vi "append at intervals.vi"(6 "Log Period [s]":dbl=10.0, 8 "error in (no error)":errorcluster, 9 "Array":dbl[](array[numeric]), 10 "Previous Time":timestamp, 11 "Data Log":refnum<class "data log.lvclass">) -> (0 "error constant":errorcluster, 2 "New Previous Time":timestamp, 3 "data log out":refnum<class "data log.lvclass">)   [LabVIEW 2025, in "data log.lvclass"]
uses:
  data log.lvclass
  data log.lvclass/data log.ctl
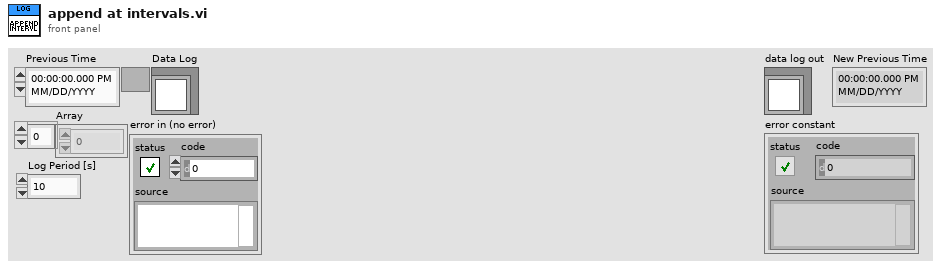
[diagram p1: front panel]
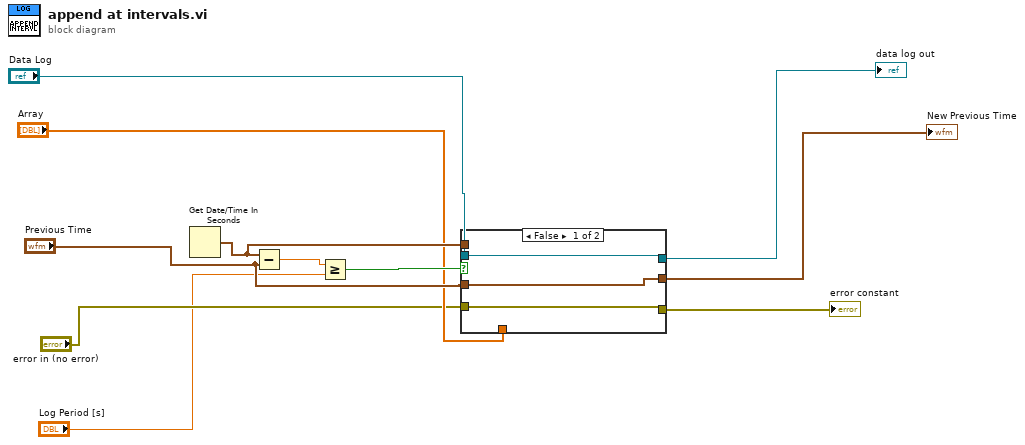
[diagram p0: block diagram]
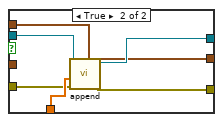
[diagram p2: hidden frame]
diagram:
  n1 = Get Date/Time In Seconds() -> (seconds since 1Jan1904=w9:timestamp)
  n2 = Subtract(x=w9, y="Previous Time") -> (x-y=w11:dbl)
  n3 = Greater Or Equal?(x=w11, y="Log Period [s]") -> (x >= y?=w10:bool)
  n4 = case shown="False" w10 {
    tunnel: [w14 w20] -> w5
    tunnel: "Data Log" -> [w14 w19]
    tunnel: "Array" -> [_ w18]
    tunnel: [w13 w17] -> w4
    tunnel: "Previous Time" -> [w13 _]
    tunnel: w9 -> [_ w17]
    tunnel: [w12 w16] -> w3
    tunnel: "error in (no error)" -> [w12 w15]
    frame False {
    }
    frame True {
      n5 = call-dynamic "append.vi"("error in (no error)"=w15, "data"=w18, "data log in"=w19) -> ("error out"=w16:errorcluster, "data log out"=w20:refnum<class "data log.lvclass">)  [unwired: 7 in]
    }
  }
  "data log out" <- w5
  "New Previous Time" <- w4
  "error constant" <- w3
